vi "ComparingTwoNumbers.vi"() -> ()   [LabVIEW 2020]
uses:
  Typedefs/EnumControl.ctl
panel:
  in  "Operations":T1
  out "Result":string
  in  "Stop":bool
  out "Boolean Result":bool
  in  "A":dbl
  in  "B":dbl
  # "Comparision of two numbers"
  # "This vi helps to check wheather two numbers statisfies the condition or not."
  # "Operation selector"
  # "Output"
  # "Input"
  # "Indicates wheather they statisfies the condition or not."
  # "Here the input number were given."
  # "Use this button to stop the conversion"
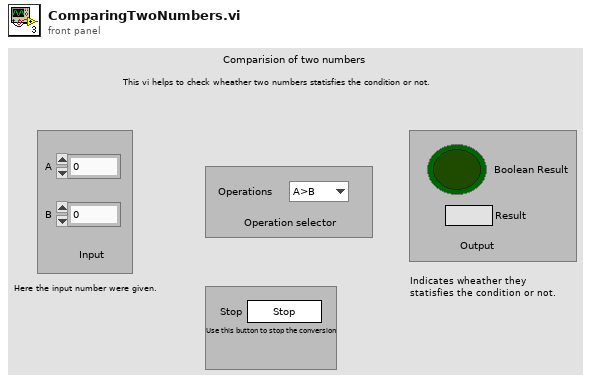
[diagram p1: front panel]
types:
  T1 = typedef "EnumControl.ctl" = enum16{"A>B", "A<B", "A>=B", "A<=B", "A=B", "A!=B"}
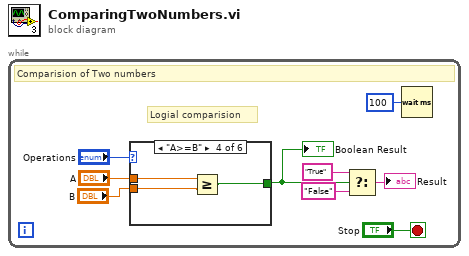
[diagram p0: block diagram]
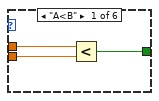
[diagram p2: hidden frame]
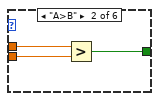
[diagram p3: hidden frame]
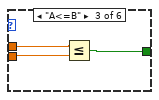
[diagram p4: hidden frame]
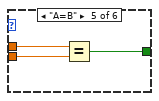
[diagram p5: hidden frame]
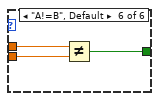
[diagram p6: hidden frame]
diagram:
  n1 = while {
    stop <- "Stop" stop-if-true
    # "Logial comparision"
    # "Comparision of Two numbers"
    n2 = case shown="\"A>=B\"" "Operations" {
      tunnel: "A" -> [w10 w14 w17 w20 w22 w25]
      tunnel: "B" -> [w11 w13 w16 w19 w23 w26]
      tunnel: [w12 w15 w18 w21 w24 w27] -> w6
      frame "A<B" {
        n3 = Less?(x=w10, y=w11) -> (x < y?=w12:bool)
      }
      frame "A>B" {
        n4 = Greater?(x=w14, y=w13) -> (0:w15:bool)
      }
      frame "A<=B" {
        n5 = Less Or Equal?(x=w17, y=w16) -> (x <= y?=w18:bool)
      }
      frame "A>=B" {
        n6 = Greater Or Equal?(x=w20, y=w19) -> (x >= y?=w21:bool)
      }
      frame "A=B" {
        n7 = Equal?(x=w22, y=w23) -> (x = y?=w24:bool)
      }
      frame "A!=B", Default {
        n8 = Not Equal?(x=w25, y=w26) -> (x != y?=w27:bool)
      }
    }
    "Boolean Result" <- w6
    n9 = Select(t="True", s=w6, f="False") -> (s? t:f=→"Result":string)
    n10 = Wait (ms)(milliseconds to wait=u32 100) -> ()  [unwired: 1 out]
  }
